vi "Save time file.vi"(8 "error in (no error)":errorcluster, 9 "File name":string="dato", 10 "prompt":string, 11 "Time chart":cluster{"Time":dbl, "Data":dbl}[](array[cluster])) -> (0 "error out":errorcluster)   [LabVIEW 2020]
uses:
  <vilib>/Utility/sysdir.llb/System Directory Type.ctl
panel:
  out "String":string
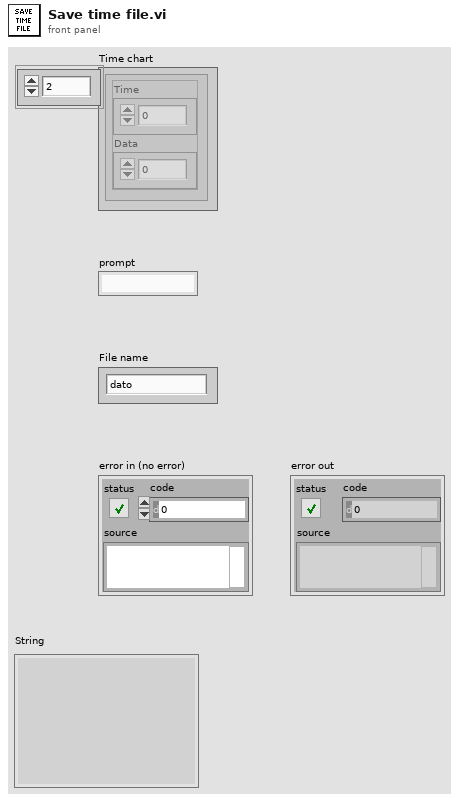
[diagram p1: front panel]
types:
  T1 = enum16{"open", "replace", "create", "open or create", "replace or create", "replace or create with confirmation"}
  T2 = typedef "System Directory Type.ctl" = i32
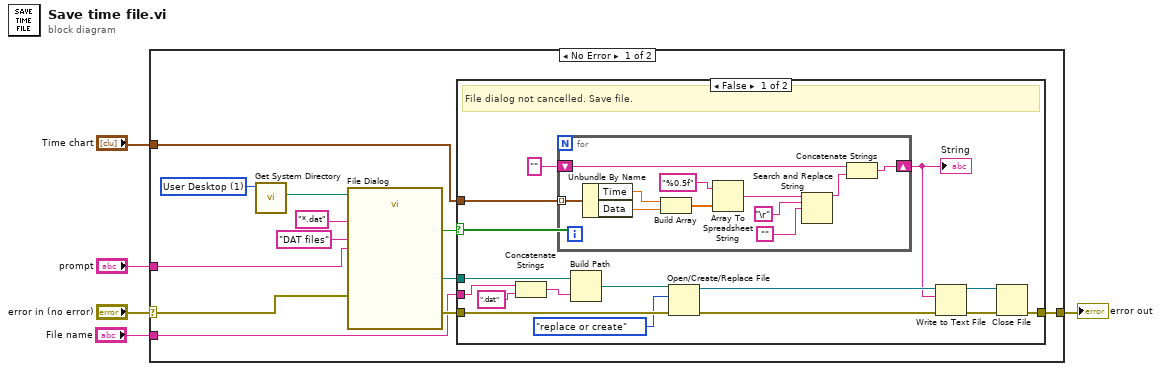
[diagram p0: block diagram]
diagram:
  n1 = case shown="No Error" "error in (no error)" {
    selector: "error in (no error)" -> [w17 w45]
    tunnel: [w11 w45] -> w4
    tunnel: "Time chart" -> [w10 _]
    tunnel: "prompt" -> [w7 _]
    tunnel: "File name" -> [w6 _]
    frame No Error {
      w16 = T2 1 items=["User Home"=0, "User Desktop"=1, "User Documents"=2, "User Application Data"=3, "User Preferences"=4, "User Temporary"=5, "Public Documents"=6, "Public Application Data"=7, "Public Preferences"=8, "Public Cache"=13, "System Core Libraries"=9, "System Installed Libraries"=10, "Application Files"=11, "Boot Volume Root"=12] ("system directory type")
      n2 = call <vilib>:"Get System Directory.vi"("system directory type"=w16) -> ("system directory"=w15:path)  [unwired: 10 in]
      n3 = call "File Dialog"("start path"=w15, "prompt"=w7, "error in"=w17, "pattern (all files)"="*.dat" ("pattern label"), "pattern label"="DAT files") -> ("selected path"=w9:path, "cancelled"=w12:bool, "error out"=w13:errorcluster)  [unwired: 7 in, 1 out]
      n4 = case shown="False" w12 {
        tunnel: w13 -> [w30 w44]
        tunnel: [w25 w44] -> w11
        tunnel: w10 -> [w32 _]
        tunnel: w9 -> [w22 _]
        tunnel: w6 -> [w20 _]
        frame False {
          # "File dialog not cancelled. Save file."
          n5 = Concatenate Strings(w20, ".dat" ("string")) -> (w18:string)
          n6 = for {
            tunnel: w32 -> [w43] mode=indexing
            shift-right: [w37] -> w26
            shift-left: "" -> [w38]
            n7 = Unbundle By Name(w43) -> ("Time"=w41:dbl, "Data"=w40:dbl)
            n8 = Build Array(w41, w40) -> (w39:dbl[])
            n9 = Array To Spreadsheet String(array=w39, 3:"%0.5f" ("format string")) -> (spreadsheet string=w36:string)  [unwired: 1 in]
            n10 = Search and Replace String(input string=w36, search string="\r", replace string="") -> (result string=w35:string)  [unwired: 5 in, 3 out]
            n11 = Concatenate Strings(w38, w35) -> (w37:string)
          }
          "String" <- w26
          n12 = Build Path(base path=w22, name or relative path=w18) -> (appended path=w21:path)
          n13 = Open/Create/Replace File(file path (use dialog)=w21, error in=w30, operation (0:open)=T1."replace or create") -> (refnum out=w27:refnum<file>, error out=w29:errorcluster)  [unwired: 3 in, 1 out]
          n14 = Write to Text File(file (use dialog)=w27, text=w26, error in=w29) -> (refnum out=w24:refnum<file>, error out=w28:errorcluster)  [unwired: 1 in, 1 out]
          n15 = Close File(refnum=w24, error in=w28) -> (error out=w25:errorcluster)  [unwired: 1 out]
        }
        frame True {
          # "Dialog cancelled. Do nothing."
        }
      }
    }
    frame Error {
    }
  }
  "error out" <- w4
